vi "Overall_system_A0-1_Weightfirst.vi"() -> ()   [LabVIEW 2019]
doc: "This VI is th overall VI that can read the weight, rfid and camera (and save the data into a csv file). When certain threshold are met it can also send a telegram message at the end."
uses:
  dependencies/notification/Telegram-Bot-master (1)/Telegram-Bot-master/Telegram/Methods/TypeDefs/SendMessageType.ctl
panel:
  out "Rfid 2":string
  in  "RFID VISA resource name 2":refnum<visa-resource-name>="COM18"
  out "Rfid":string
  in  "RFID VISA resource name":refnum<visa-resource-name>="COM5"
  in  "start condition (debug)":bool
  out "Weight":string
  in  "delay before read (ms)":u32=500
  in  "Weight VISA resource name":refnum<visa-resource-name>="COM1"
  in  "start rfid (debug)":bool
  in  "Start camera (debug)":bool
  out "Health Monitoring in Progress":bool
  in  "Bird is underfeeding (debug)":bool
  out "Current image":T1(plugin-control)
  in  "Camera Name":refnum<k21>="cam0" caption="IMAQdx Session"
  # "Intelligent Health Monitoring System"
  # "grams"
  # "Weight detection settings:"
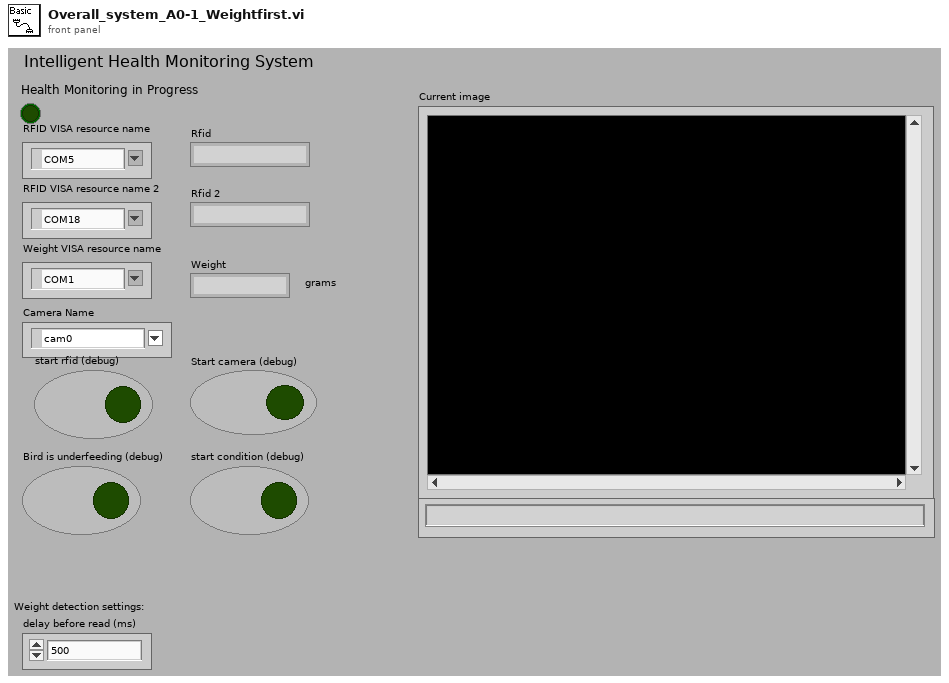
[diagram p1: front panel]
types:
  T1 = typedef "IMAQ Image.ctl" = refnum<image>
  T2 = typedef "SendMessageType.ctl" = enum16{"Text", "ReplyKeyboardMarkup", "ReplyKeyboardRemove"}
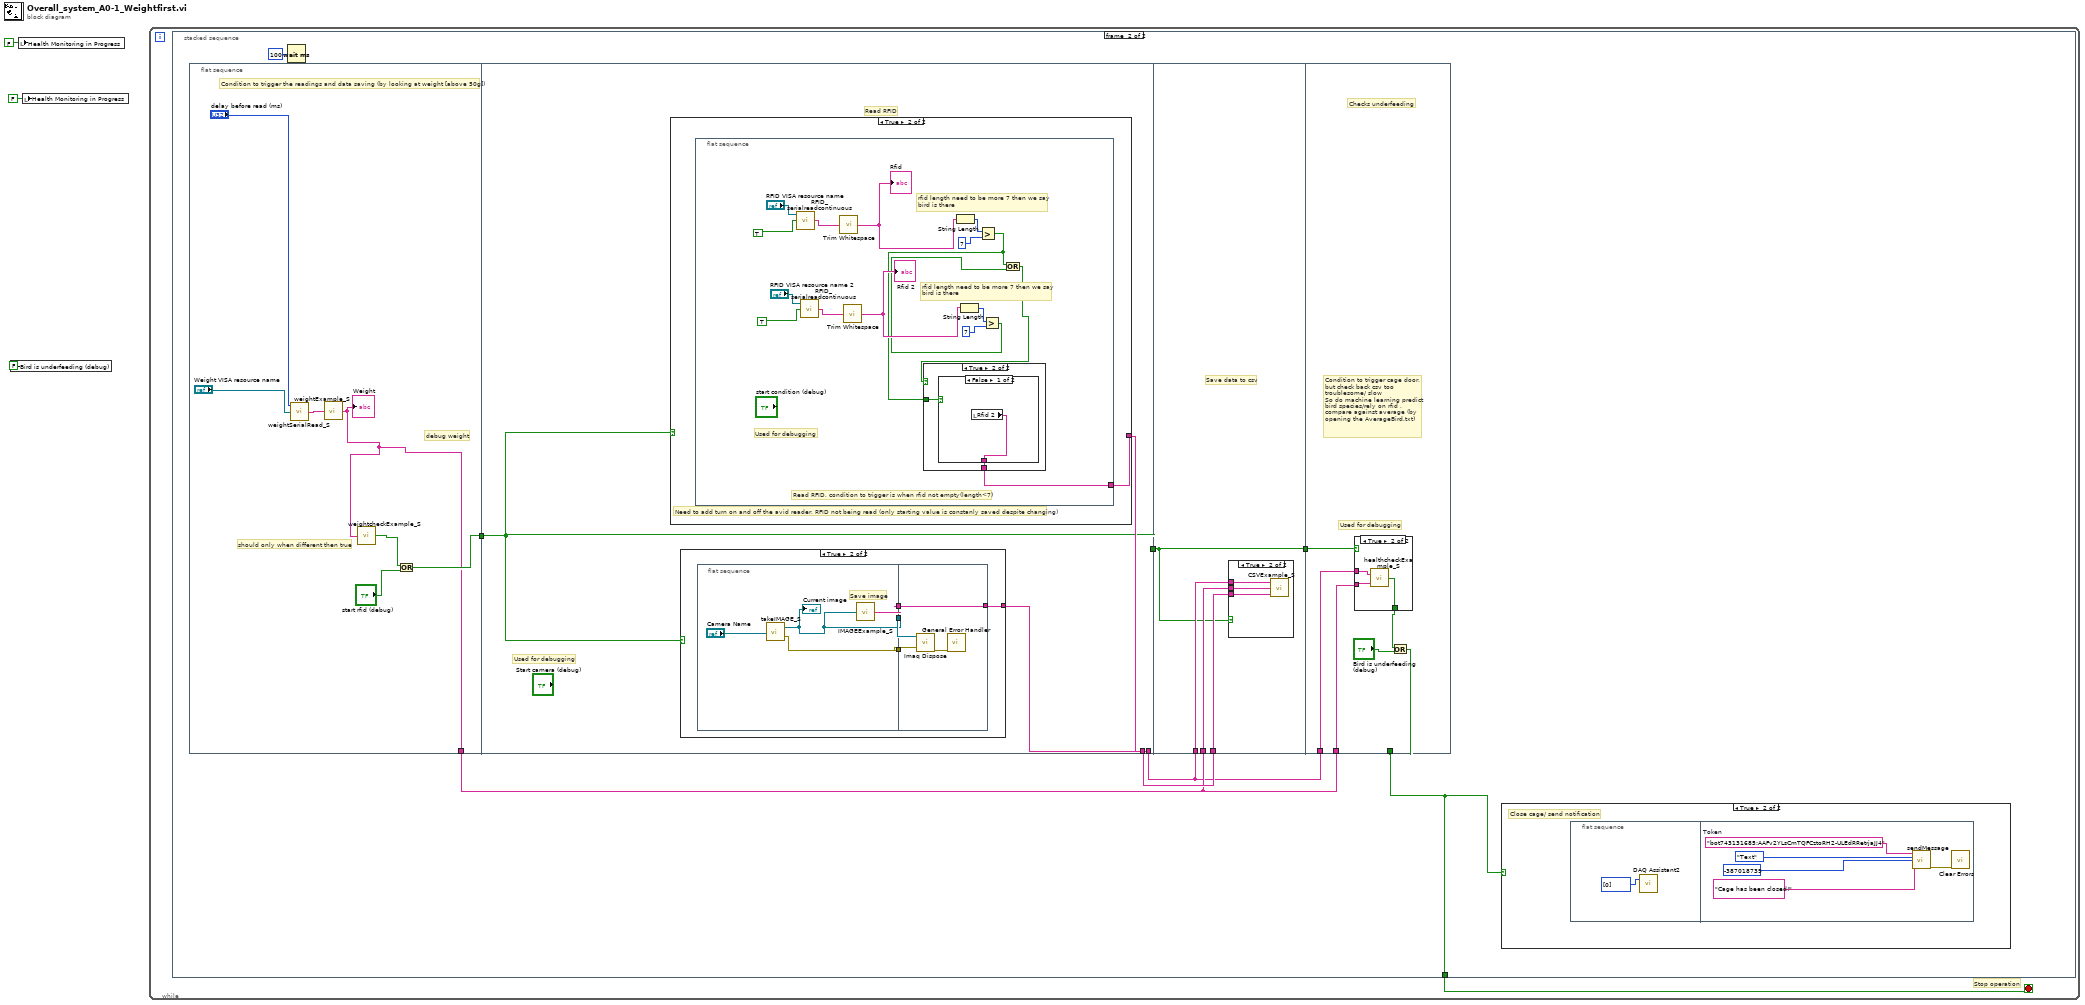
[diagram p0: block diagram]
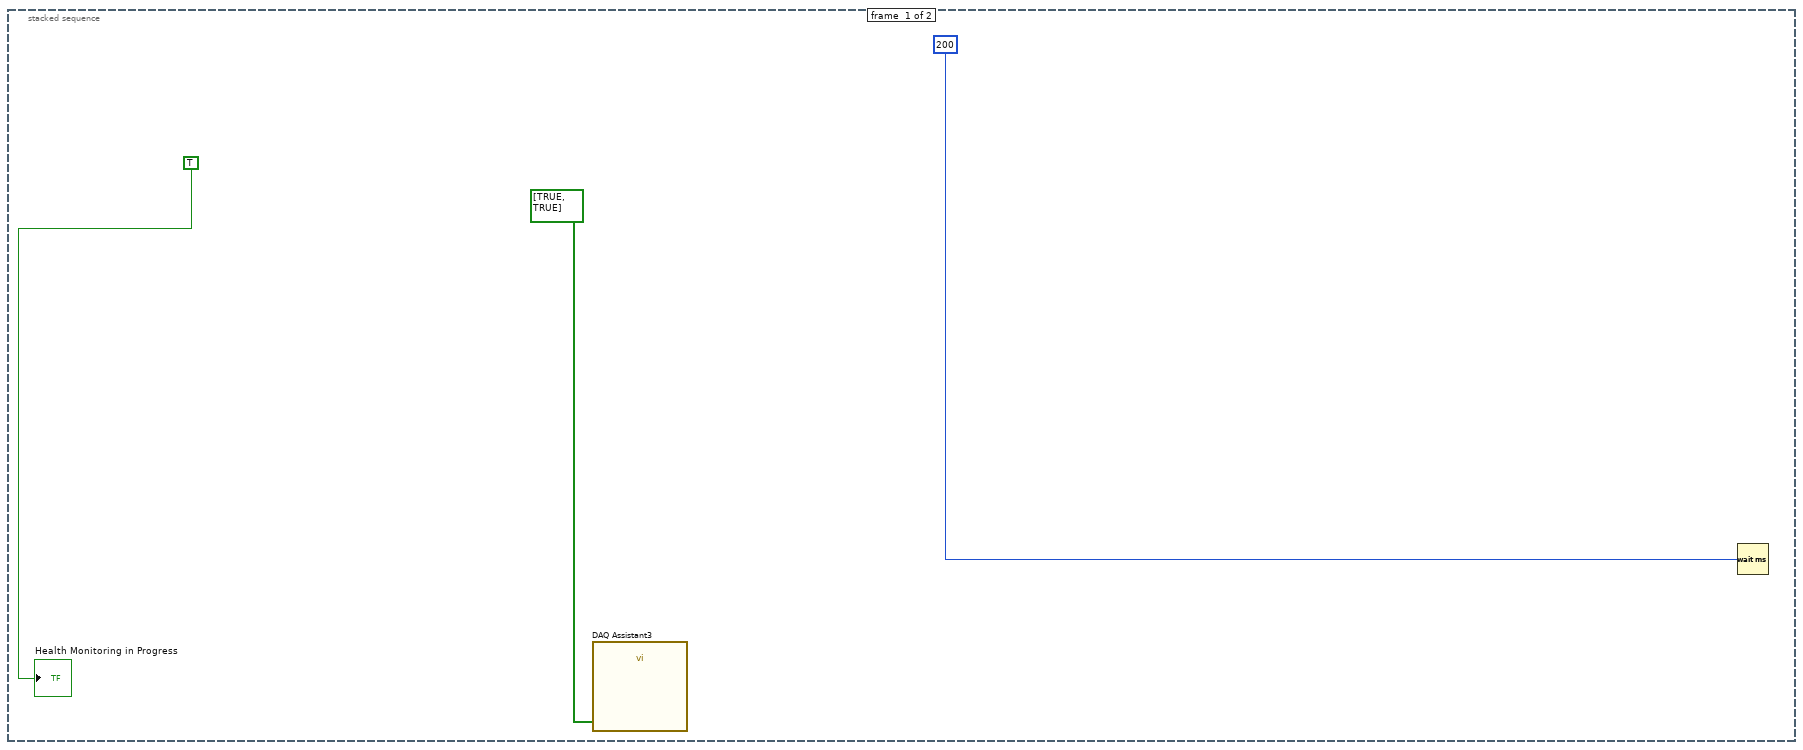
[diagram p2: hidden frame]
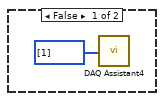
[diagram p4: hidden frame]
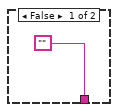
[diagram p5: hidden frame]
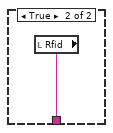
[diagram p6: hidden frame]
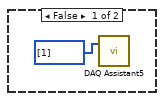
[diagram p9: hidden frame]
diagram:
  n1 = local write "Bird is underfeeding (debug)"(FALSE ("Bird is underfeeding")) -> ()
  n2 = local write "Health Monitoring in Progress"(FALSE ("Health Monitoring in Progress")) -> ()
  n3 = local write "Health Monitoring in Progress"(FALSE ("Health Monitoring in Progress")) -> ()
  n4 = while {
    stop <- w4 stop-if-true
    # "Stop operation"
    n5 = stacked-sequence {
      tunnel: [_ w14] -> w4
      frame #0 {
        n6 = call "DAQ Assistant3"("data"=bool[] [TRUE, TRUE]) -> ()  [unwired: 17 in, 2 out]
        n7 = Wait (ms)(milliseconds to wait=u32 200) -> ()  [unwired: 1 out]
        "Health Monitoring in Progress" <- TRUE ("Health Monitoring in Progress")
      }
      frame #1 {
        n8 = flat-sequence {
          tunnel: [w16] -> w9
          tunnel: [w21] -> w13
          tunnel: [w25] -> w8
          tunnel: [w24] -> w10
          tunnel: w13 -> [w23]
          tunnel: [w23] -> w12
          tunnel: w12 -> [w61]
          tunnel: [w61] -> w11
          tunnel: w10 -> [w64]
          tunnel: w9 -> [w63]
          tunnel: w8 -> [w62]
          tunnel: [w68] -> w14
          tunnel: w9 -> [w73]
          tunnel: w11 -> [w72]
          tunnel: w8 -> [w71]
          frame #0 {
            # "debug weight"
            # "Condition to trigger the readings and data saving (by looking at weight [above 50g])"
            # "should only when different then true"
            n9 = call "weightSerialRead_S.vi"("Weight VISA resource name"="Weight VISA resource name", "delay before read (ms)"="delay before read (ms)") -> ("String"=w19:string)  [unwired: 1 in]
            n10 = call "weightExample_S.vi"("weight"=w19) -> ("String"=w16:string)
            "Weight" <- w16
            n11 = call "weightcheckExample_S.vi"("weight"=w16) -> ("Boolean"=w20:bool)
            n12 = Or(x=w20, y="start rfid (debug)") -> (x .or. y?=w21:bool)
          }
          frame #1 {
            # "Used for debugging"
            # "Read RFID"
            n13 = case shown="True" w23 {
              tunnel: [_ w39] -> w25
              frame False {
                n14 = call "DAQ Assistant4"("data"=u32[] [1]) -> ()  [unwired: 17 in, 2 out]
              }
              frame True {
                # "Need to add turn on and off the avid reader, RFID not being read (only starting value is constanly saved despite changing)"
                n15 = flat-sequence {
                  tunnel: [w40] -> w39
                  frame #0 {
                    # "rfid length need to be more 7 then we say \nbird is there"
                    # "Used for debugging"
                    # "rfid length need to be more 7 then we say \nbird is there"
                    # "Read RFID, condition to trigger is when rfid not empty(length<7)"
                    n16 = call "RFID_serialreadcontinuous.vi"("Read 2"=TRUE, "VISA resource name"="RFID VISA resource name") -> ("Response 2"=w52:string)  [unwired: 1 in]
                    n17 = call "RFID_serialreadcontinuous.vi"("Read 2"=TRUE, "VISA resource name"="RFID VISA resource name 2") -> ("Response 2"=w47:string)  [unwired: 1 in]
                    n18 = call <vilib>:"Trim Whitespace.vi"("string"=w52) -> ("trimmed string"=w53:string)  [unwired: 1 in]
                    "Rfid" <- w53
                    n19 = call <vilib>:"Trim Whitespace.vi"("string"=w47) -> ("trimmed string"=w48:string)  [unwired: 1 in]
                    "Rfid 2" <- w48
                    n20 = String Length(string=w53) -> (length=w55:i32)
                    n21 = String Length(string=w48) -> (length=w49:i32)
                    n22 = Greater?(x=w55, y=7) -> (0:w41:bool)
                    n23 = Greater?(x=w49, y=7) -> (0:w43:bool)
                    n24 = Or(x=w41, y=w43) -> (x .or. y?=w42:bool)
                    n25 = case shown="True" w42 {
                      tunnel: w41 -> [_ w58]
                      tunnel: ["" w57] -> w40
                      frame False {
                      }
                      frame True {
                        n26 = case shown="False" w58 {
                          tunnel: [w59 w60] -> w57
                          frame False {
                            n27 = local read "Rfid 2"() -> (w59:string)
                          }
                          frame True {
                            n28 = local read "Rfid"() -> (w60:string)
                          }
                        }
                      }
                    }
                  }
                }
              }
            }
            n29 = case shown="True" w23 {
              tunnel: [_ w27] -> w24
              frame False {
              }
              frame True {
                n30 = flat-sequence {
                  tunnel: [w31] -> w29
                  tunnel: [w30] -> w28
                  tunnel: [w33] -> w26
                  tunnel: w29 -> [w37]
                  tunnel: w28 -> [w35]
                  tunnel: [w34] -> w27
                  tunnel: w26 -> [w34]
                  frame #0 {
                    # "Save image"
                    n31 = call "takeIMAGE_S.vi"("Camera Name"="Camera Name") -> ("Current image"=w30:T1, "error in (no error)"=w31:errorcluster)
                    "Current image" <- w30
                    n32 = call "IMAGEExample_S.vi"("Image"=w30) -> ("String"=w33:string)
                  }
                  frame #1 {
                    n33 = call "Imaq Dispose"("Image"=w35, "error in (no error)"=w37) -> ("error out"=w36:errorcluster)  [unwired: 4 in]
                    n34 = call <vilib>:"General Error Handler.vi"("error in (no error)"=w36) -> ()  [unwired: 2 in, 13 out]
                  }
                }
              }
            }
          }
          frame #2 {
            # "Save data to csv"
            n35 = case shown="True" w61 {
              tunnel: w64 -> [_ w65]
              tunnel: w63 -> [_ w66]
              tunnel: w62 -> [_ w67]
              frame False {
              }
              frame True {
                n36 = call "CSVExample_S.vi"("imageId"=w65, "weight"=w66, "rfid"=w67) -> ()
              }
            }
          }
          frame #3 {
            # "Used for debugging"
            # "Condition to trigger cage door,\nbut check back csv too troublesome/ slow\nSo do machine learning predict bird species/rely on rfid , compare against average (by opening the AverageBird.txt)"
            # "Checks underfeeding"
            n37 = case shown="True" w72 {
              tunnel: [_ w74] -> w70
              tunnel: w71 -> [_ w75]
              tunnel: w73 -> [_ w76]
              frame False {
              }
              frame True {
                n38 = call "healthcheckExample_S.vi"("weight"=w76, "rfid"=w75) -> ("Boolean"=w74:bool)
              }
            }
            n39 = Or(x=w70, y="Bird is underfeeding (debug)") -> (x .or. y?=w68:bool)
          }
        }
        n40 = Wait (ms)(milliseconds to wait=u32 100) -> ()  [unwired: 1 out]
        n41 = case shown="True" w14 {
          frame False {
            n42 = call "DAQ Assistant5"("data"=u32[] [1]) -> ()  [unwired: 17 in, 2 out]
          }
          frame True {
            # "Close cage/ send notification"
            n43 = flat-sequence {
              frame #0 {
                n44 = call "DAQ Assistant2"("data"=u32[] [0]) -> ()  [unwired: 17 in, 2 out]
              }
              frame #1 {
                w82 = "bot743131685:AAFv2YLsCmTQFCztoRH2-ULEdRRetrjaJJ4"  # Token
                n45 = call "sendMessage.vi"("Token"=w82, "MsgType"=SendMessageType."Text", "ChatId"=i64 -387018739, "Text"="Cage has been closed!") -> ("error out"=w83:errorcluster)  [unwired: 11 in]
                n46 = call <vilib>:"Clear Errors.vi"("error in (no error)"=w83) -> ()  [unwired: 5 in, 2 out]
              }
            }
          }
        }
      }
    }
  }
